vi "ATM_Client.vi"() -> ()   [LabVIEW 2023]
uses:
  Controller/ControllerAccount.ctl
  Controller/ControllerATM.ctl
  Controller/ControllerMenu.ctl
  <vilib>/Utility/error.llb/Trim Whitespace One-Sided.vi
  <vilib>/Utility/file.llb/Read Delimited Spreadsheet (string).vi
  <vilib>/regexp/Match Regular Expression.xnode
panel:
  out "Error reading \nLog.txt":errorcluster
  out "Error reading \nAccounts.txt":errorcluster
  out "Withdrawal Error":errorcluster
  out "Deposit Error":errorcluster
  out "Fast Cash \nWithdrawal Error":errorcluster
  out "Exit Error":errorcluster
  out "Check Balance \nError":errorcluster
  out "Operation \nTimeout Error":errorcluster
  out "Login Timeout Error":errorcluster
  out "Login Error":errorcluster
  in  "Exit Admin Page":bool
  in  "Admin":enum32{"User Details", "Log Acivity"}(tab)
  out "Users":string[][](table)
  out "Log":string[][](table)
  in  "Right Buttons":T1
  out "Right Menu":T2
  out "Left Menu":T3
  in  "Left Buttons":T4
  out "Events":T5
  in  "Account No.":string
  in  "Enter Button":bool
  in  "User Input":string
  in  "Card Simulator":bool
  out "ATM Messages":string
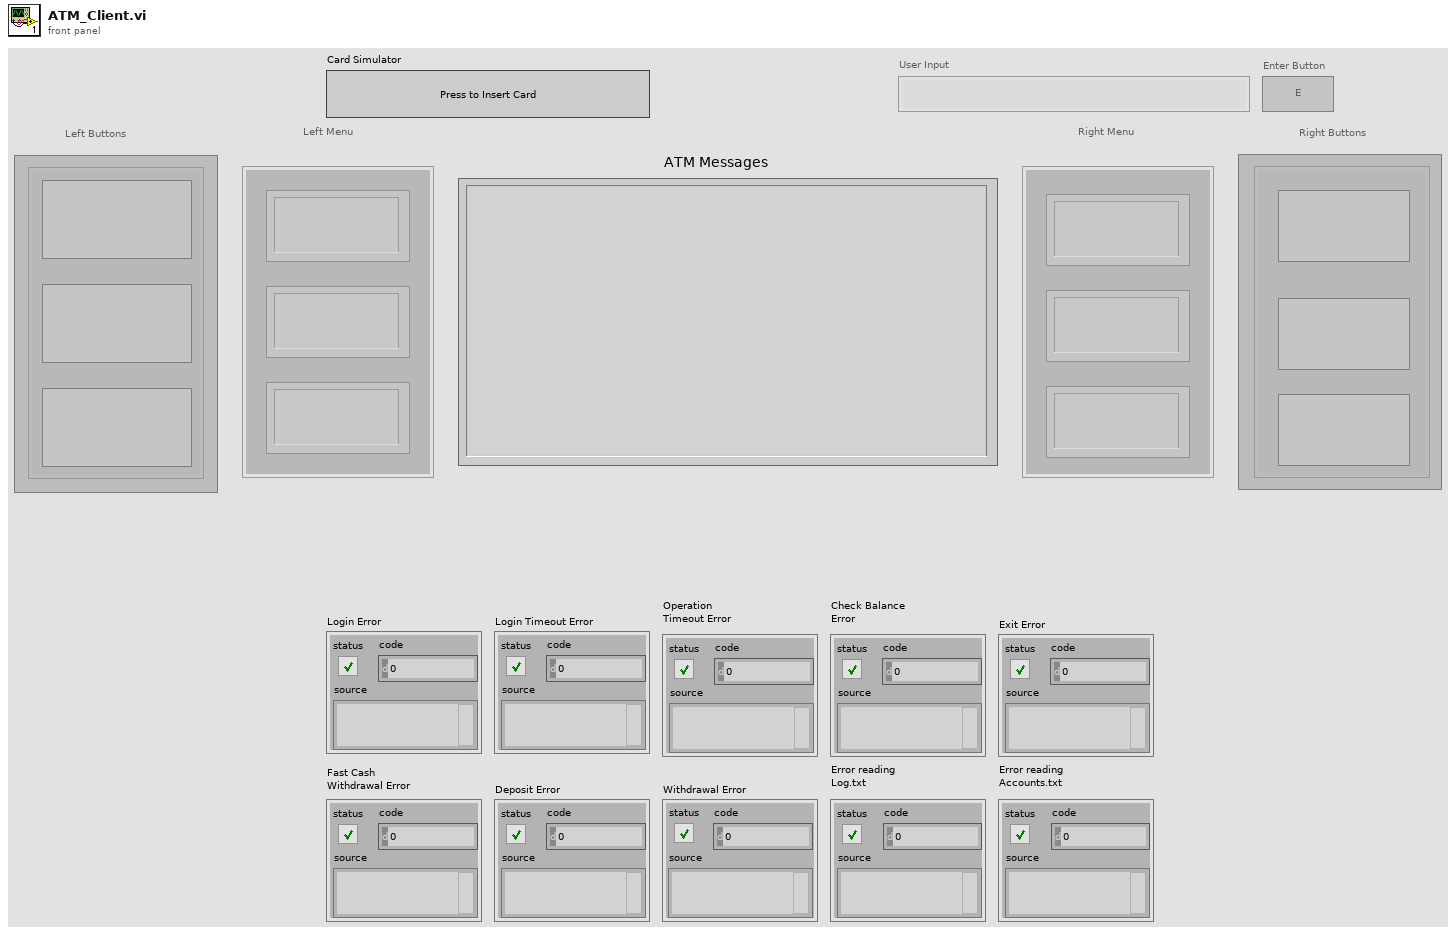
[diagram p1: front panel]
types:
  T1 = cluster{"Right Button 1":bool, "Right Button 2":bool, "Right Button 3":bool}
  T2 = cluster{"Right Menu 1":string, "Right Menu 2":string, "Right Menu 3":string}
  T3 = cluster{"Left Menu 1":string, "Left Menu 2":string, "Left Menu 3":string}
  T4 = cluster{"Left Button 1":bool, "Left Button 2":bool, "Left Button 3":bool}
  T5 = typedef "ControllerAccount.ctl" = enum16{"Deactivate", "Deposit", "Withdraw"}
  T6 = typedef "ControllerATM.ctl" = enum16{"Welcome", "Login", "Main"}
  T7 = enum8{"Enabled", "Disabled", "Disabled and Grayed Out"}
  T8 = typedef "ControllerMenu.ctl" = enum16{"Initialization", "Processes"}
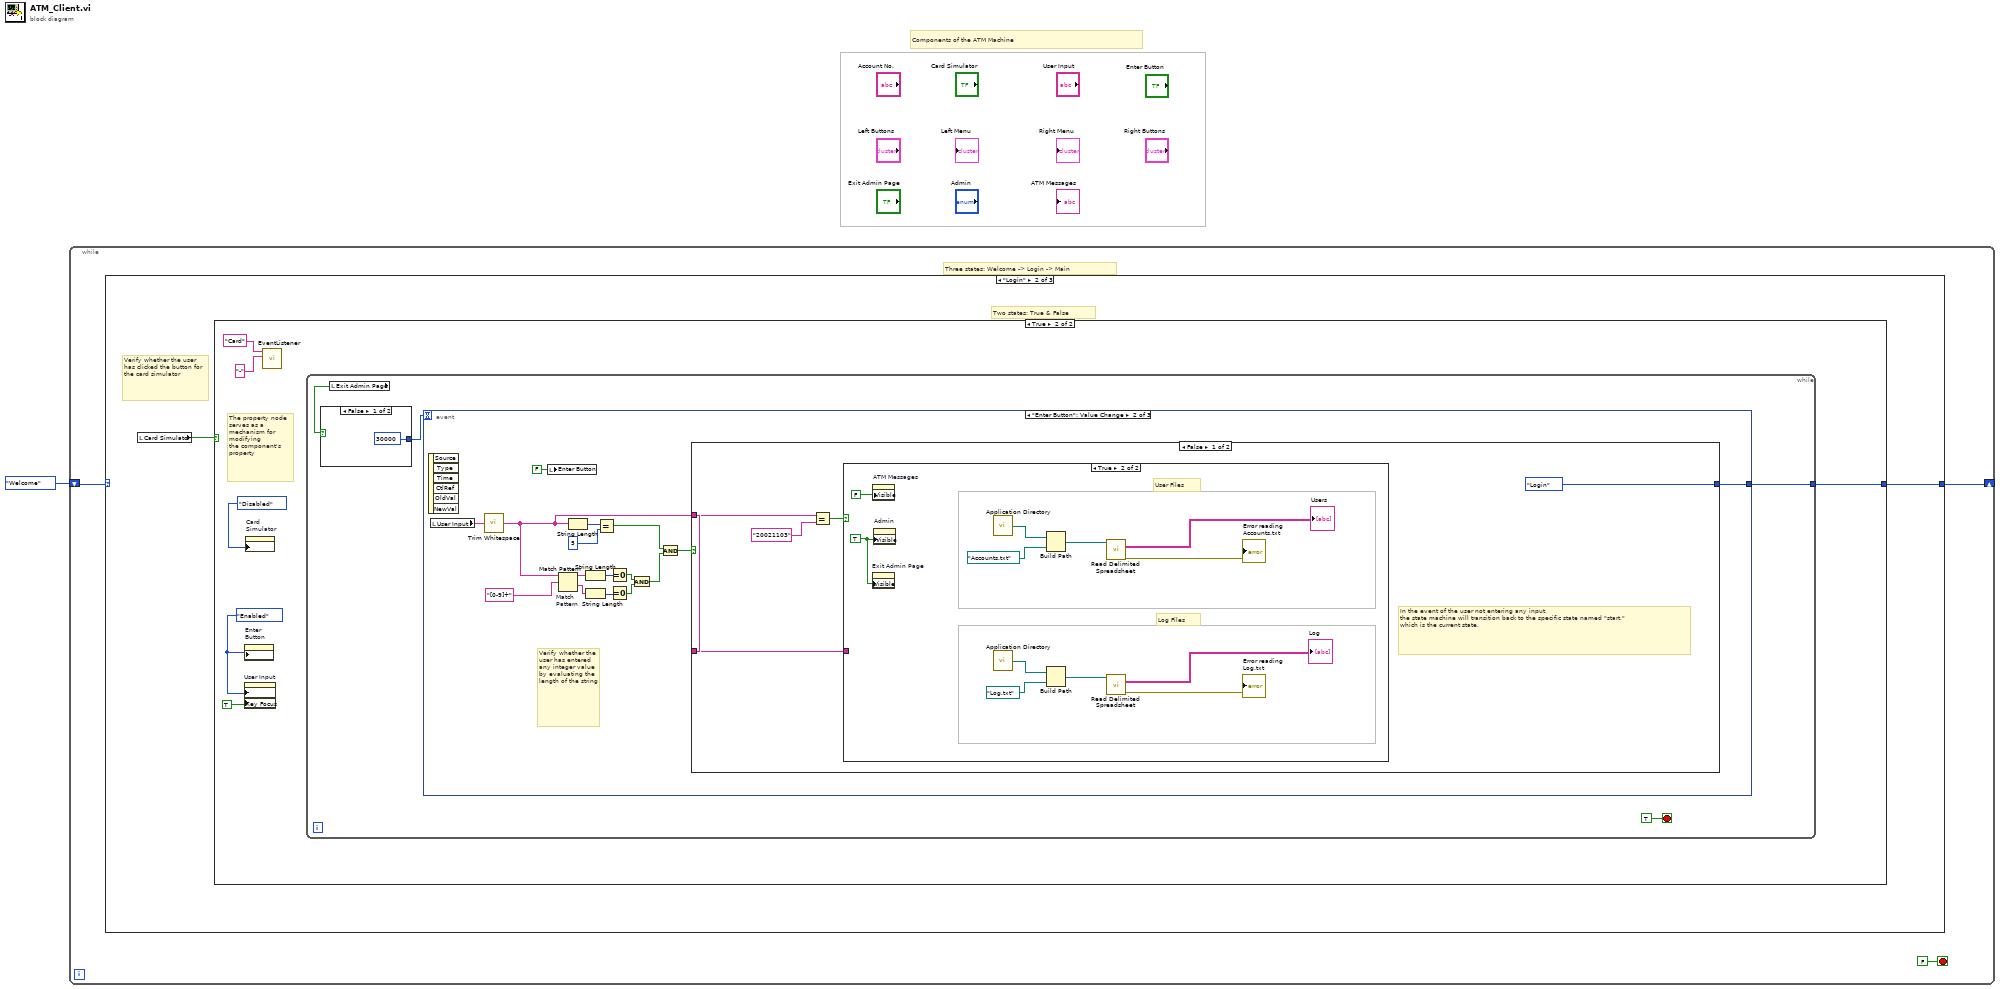
[diagram p0: block diagram]
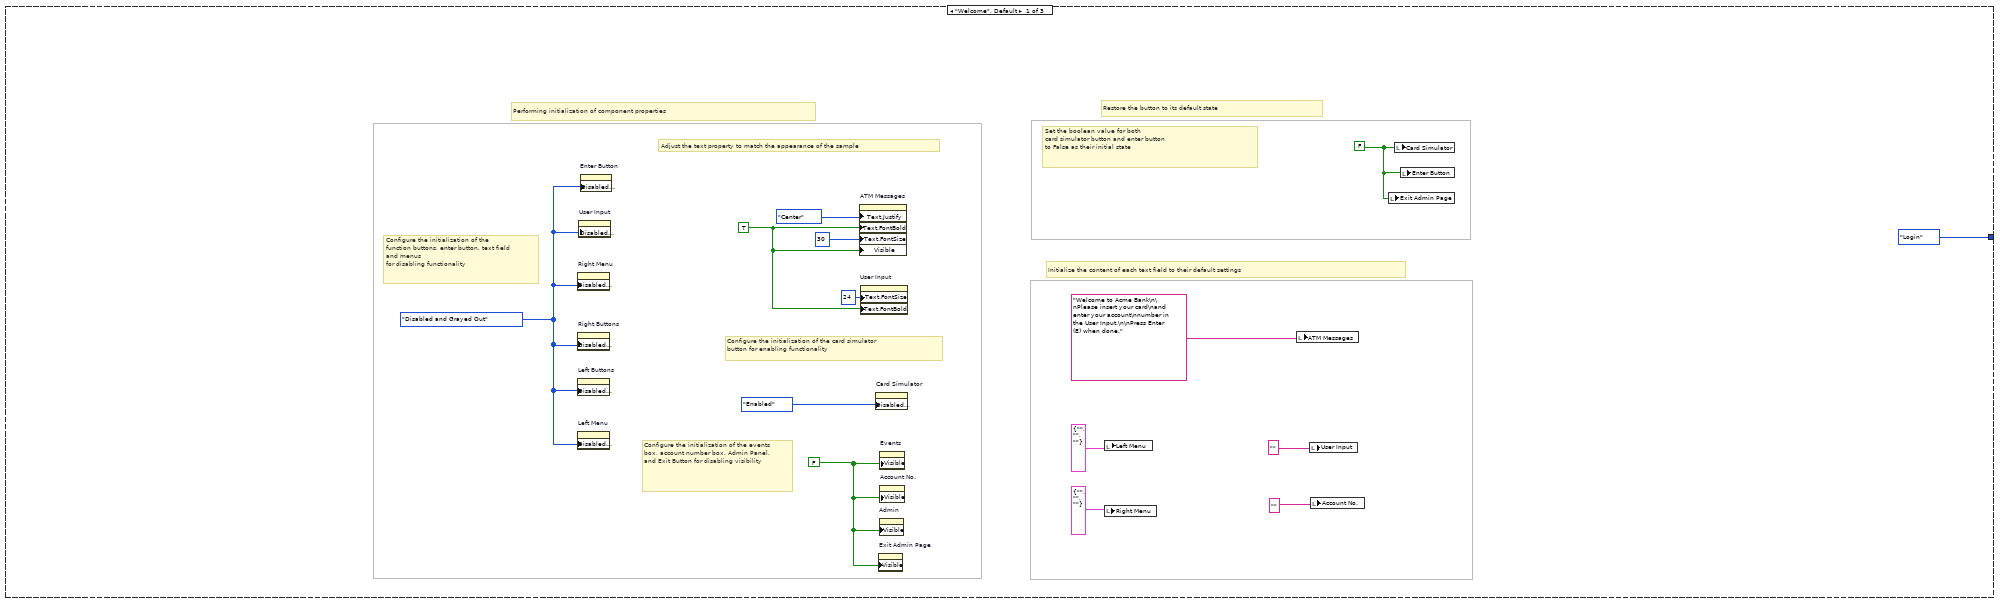
[diagram p2: hidden frame]
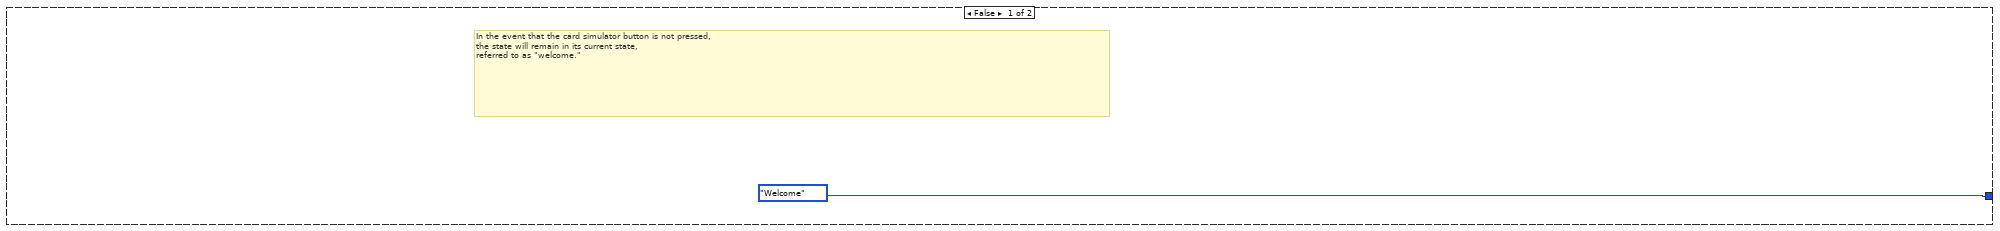
[diagram p3: hidden frame]
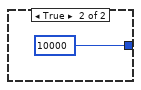
[diagram p4: hidden frame]
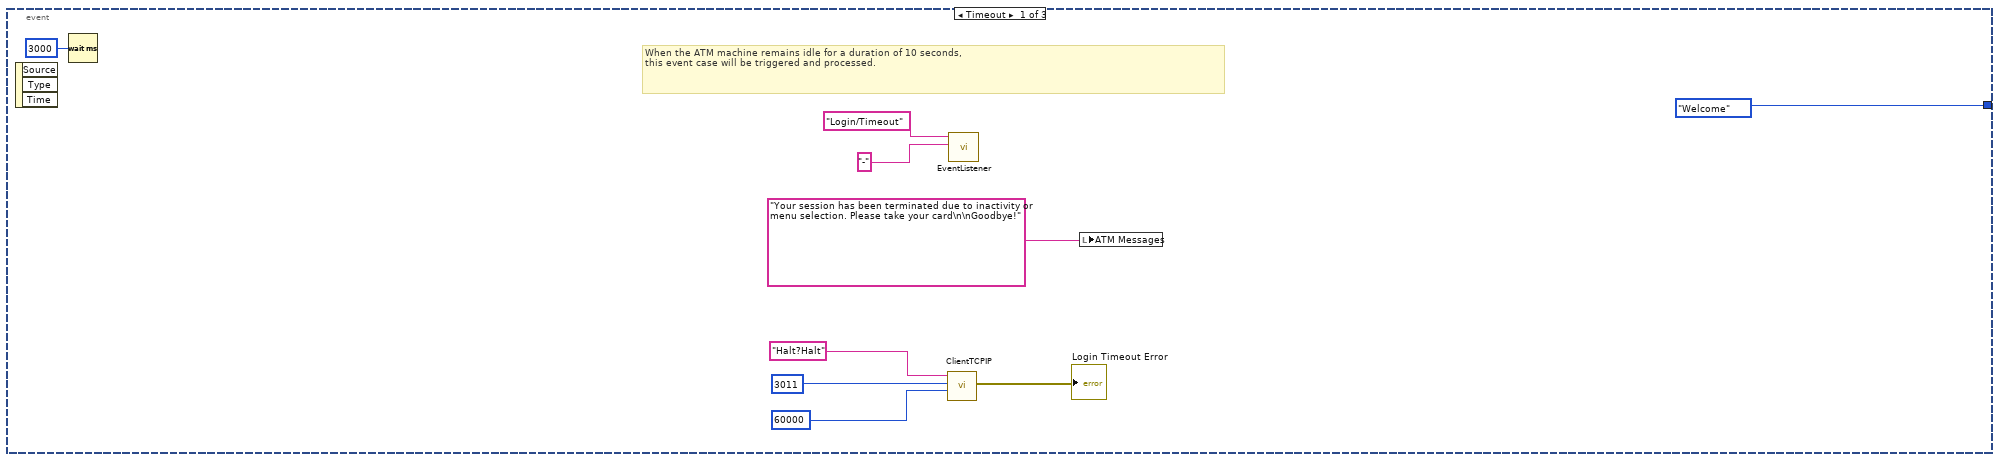
[diagram p5: hidden frame]
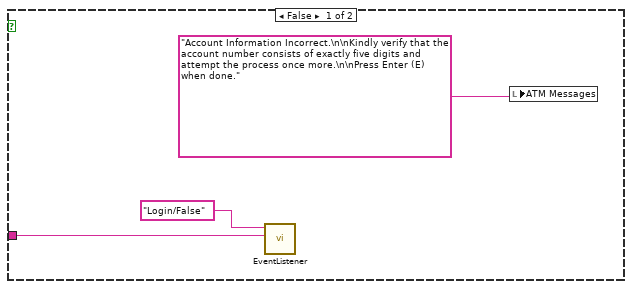
[diagram p6: hidden frame]
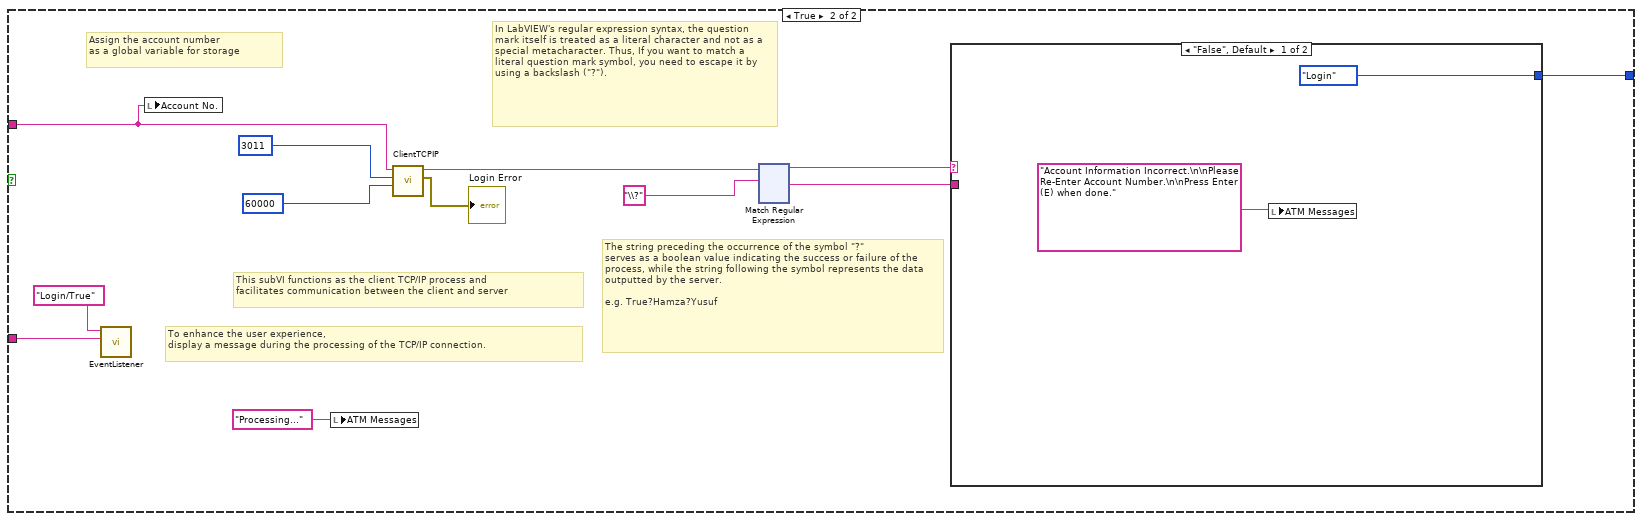
[diagram p7: hidden frame]
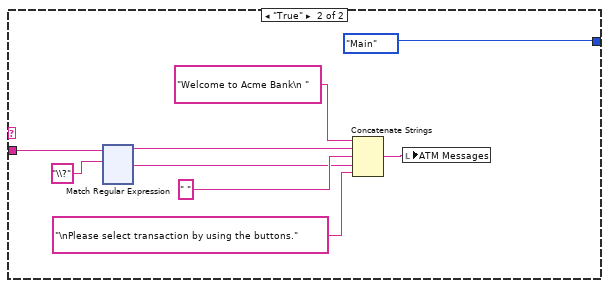
[diagram p8: hidden frame]
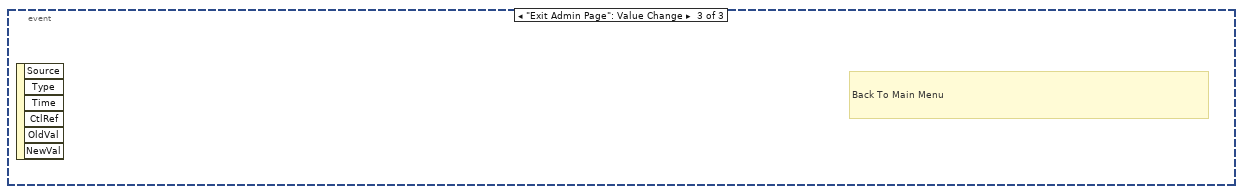
[diagram p9: hidden frame]
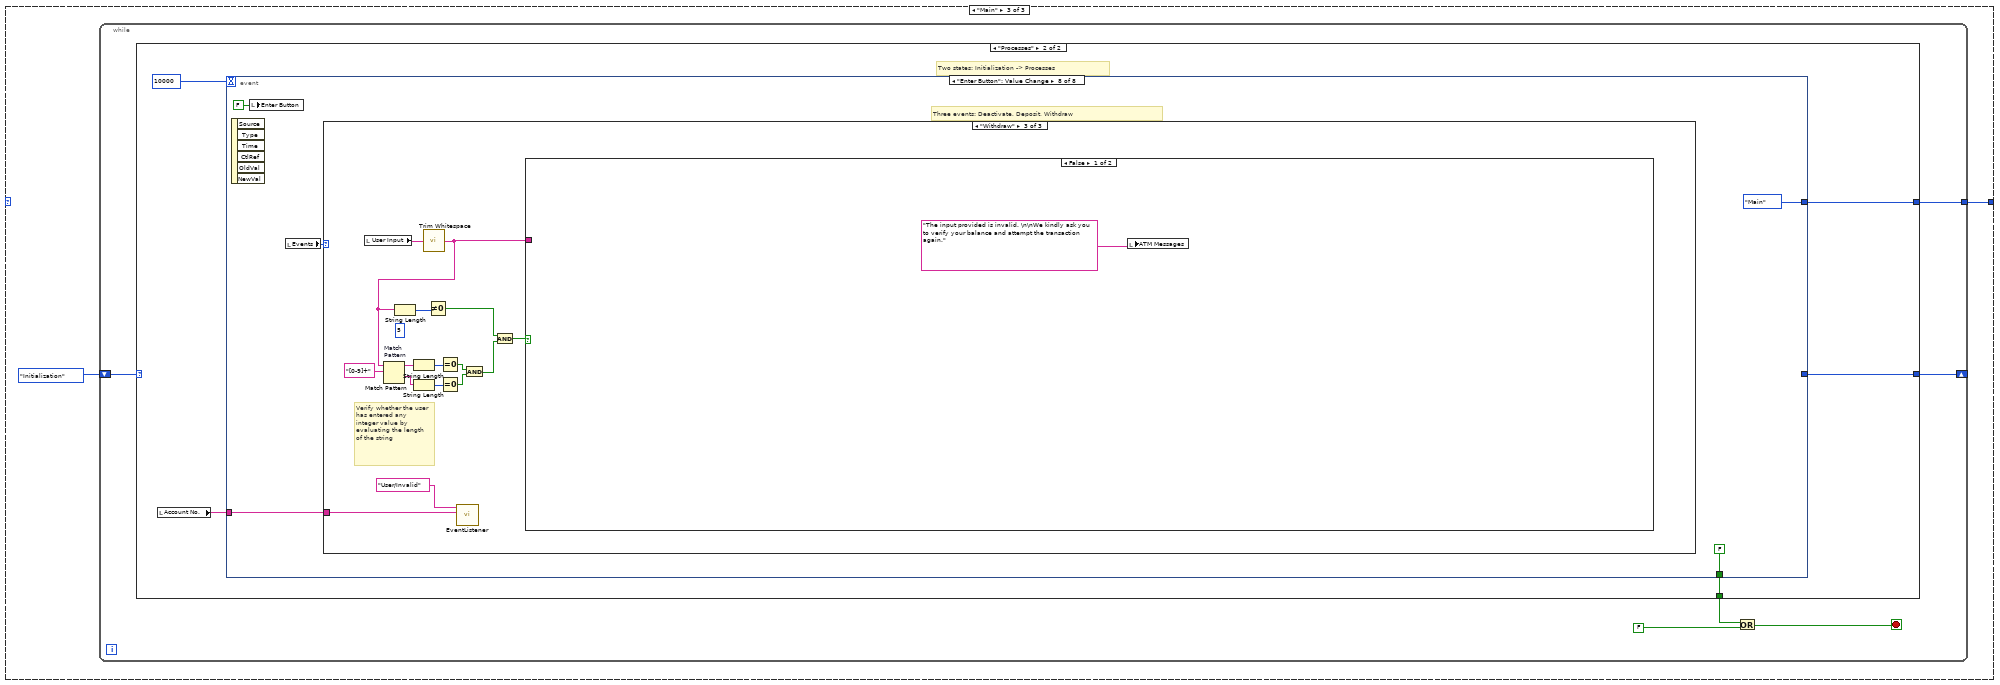
[diagram p10: hidden frame]
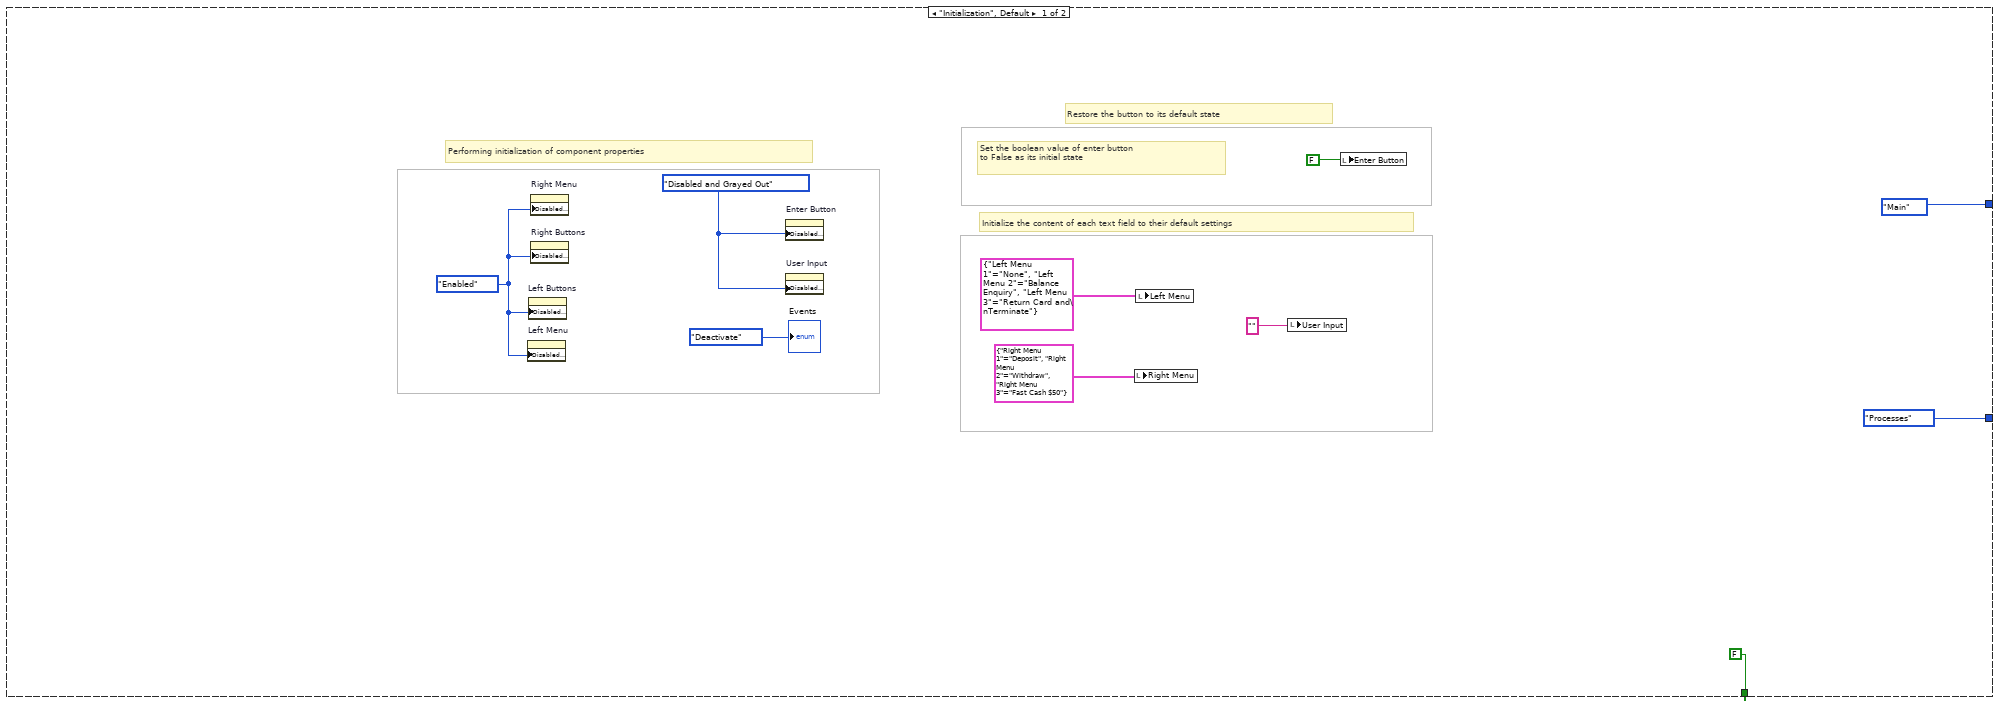
[diagram p11: hidden frame]
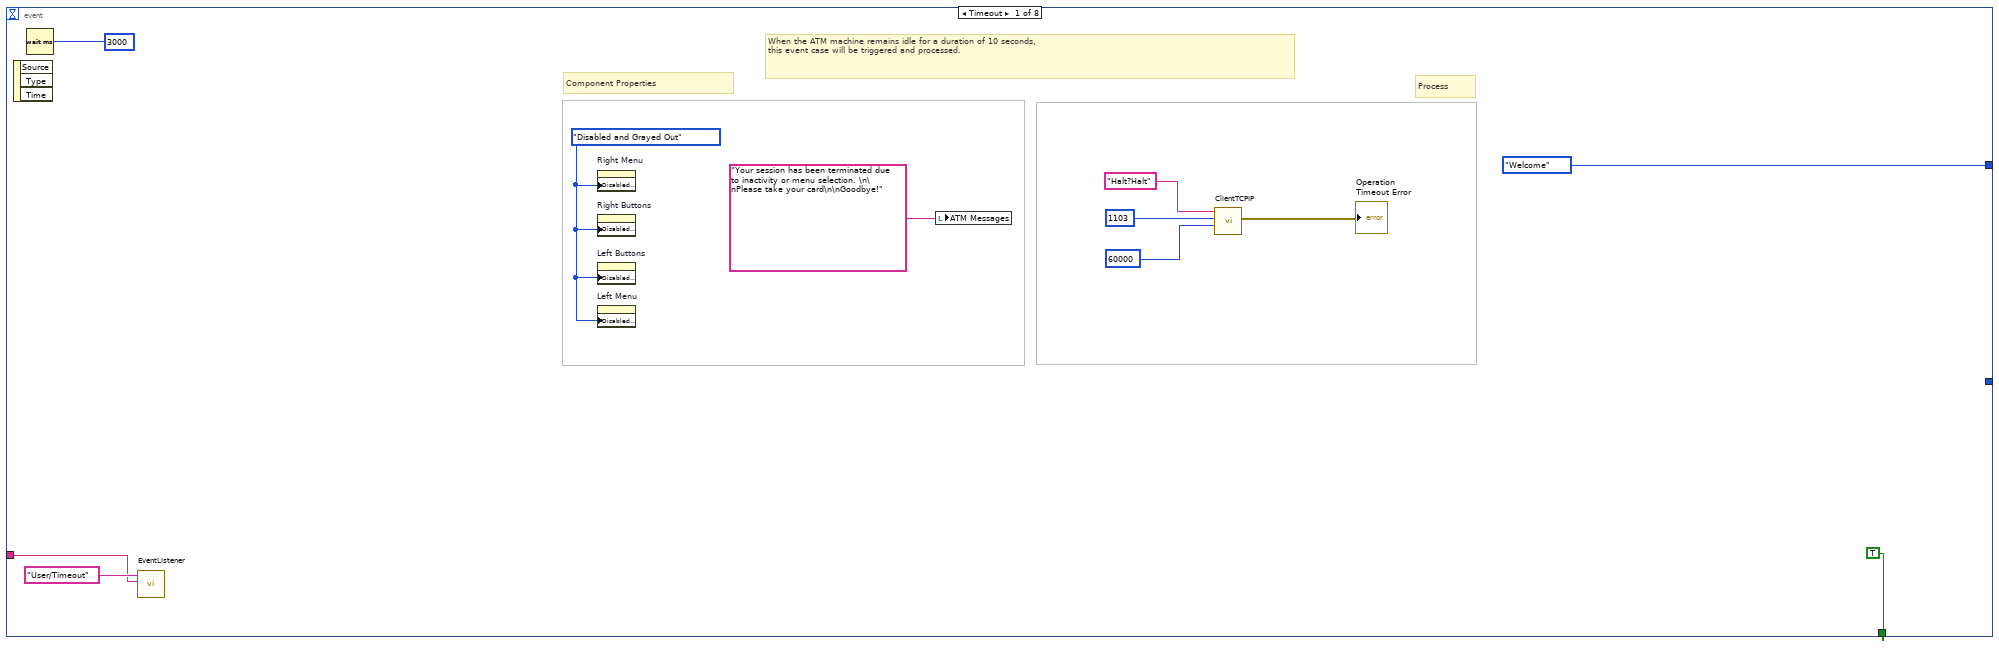
[diagram p12: hidden frame]
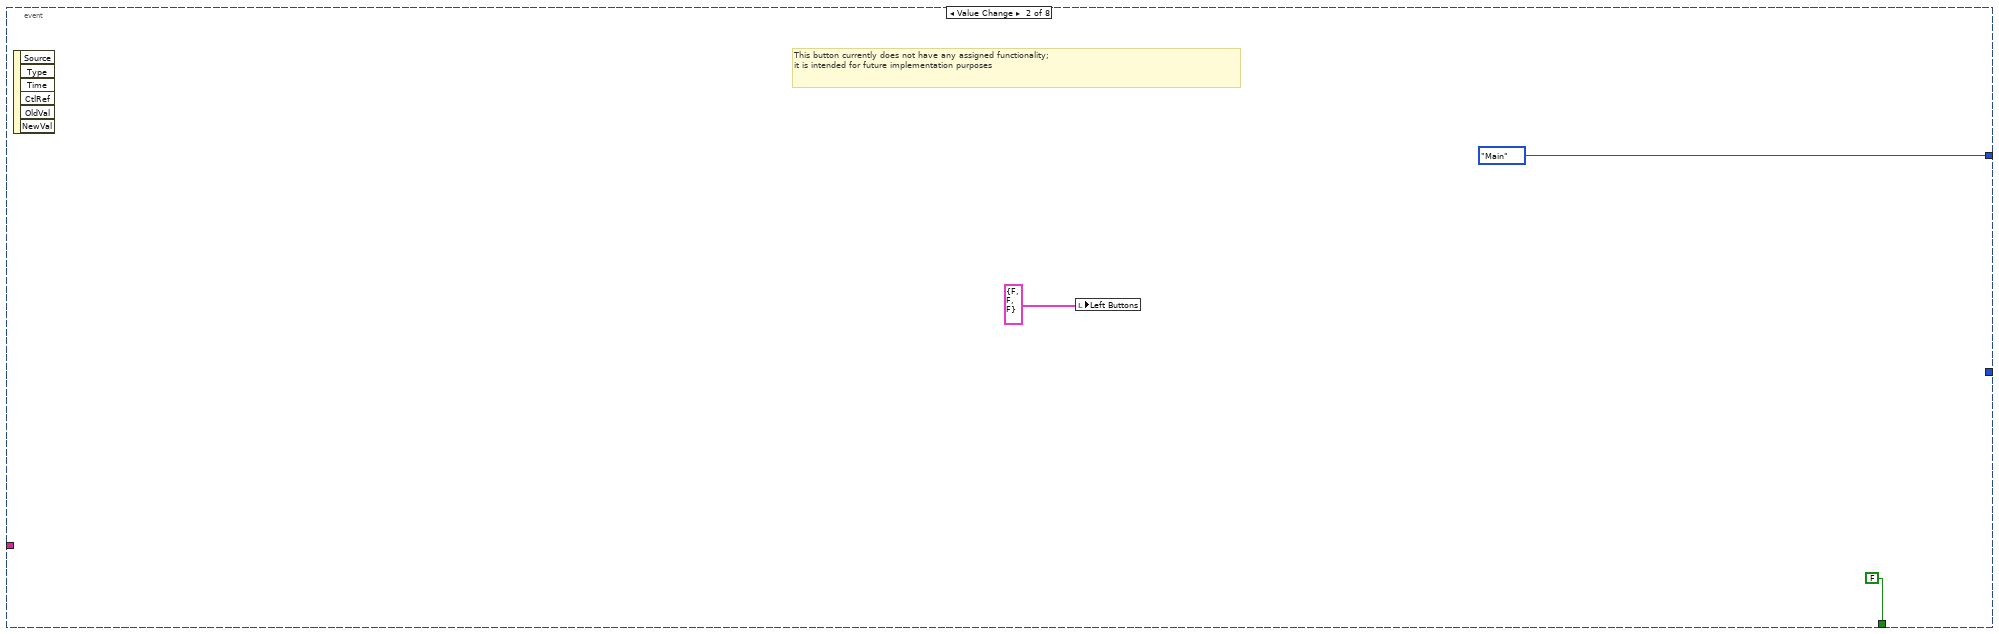
[diagram p13: hidden frame]
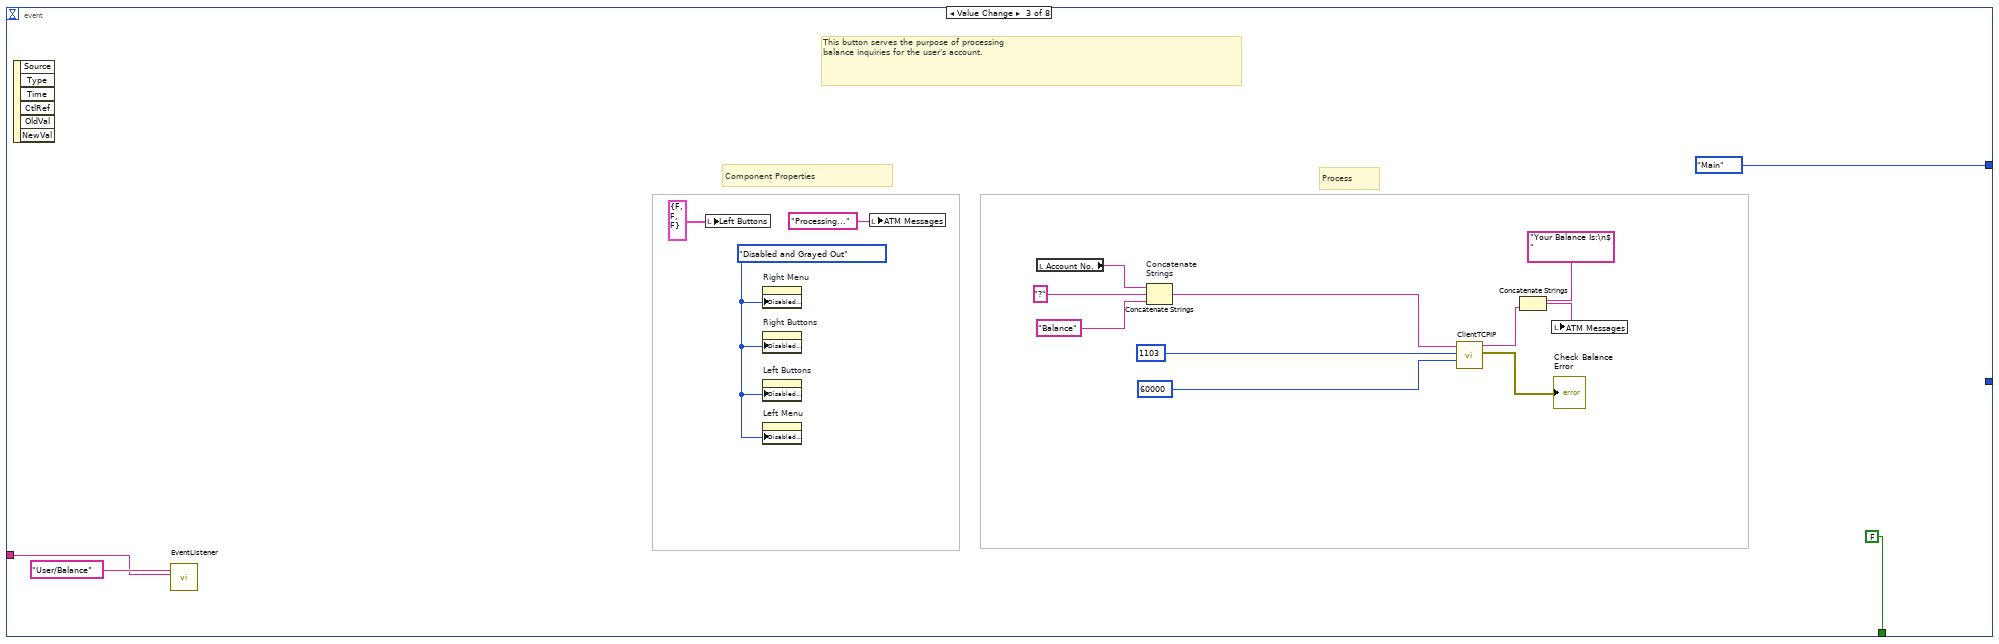
[diagram p14: hidden frame]
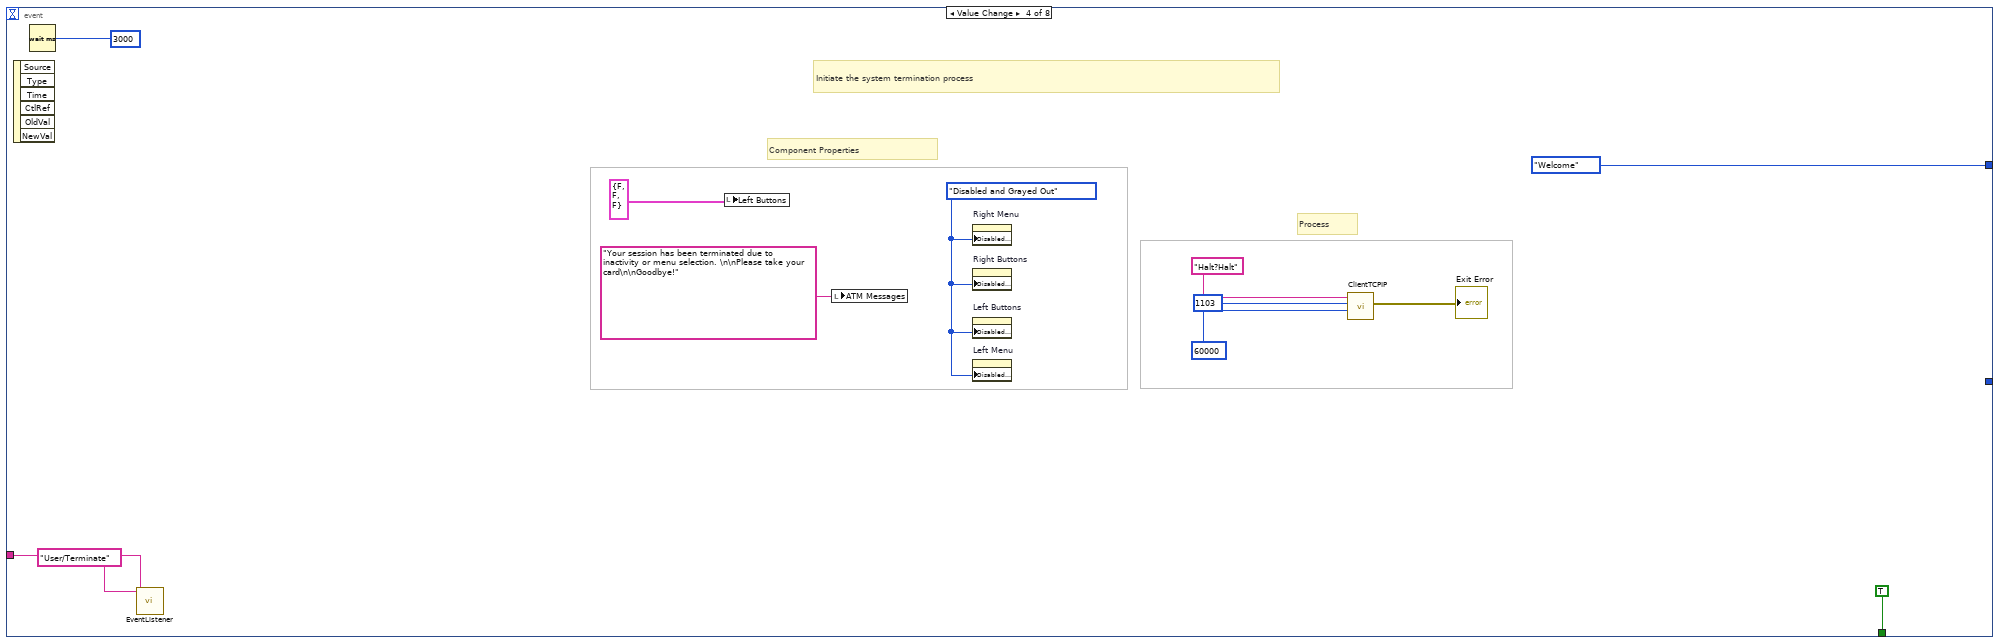
[diagram p15: hidden frame]
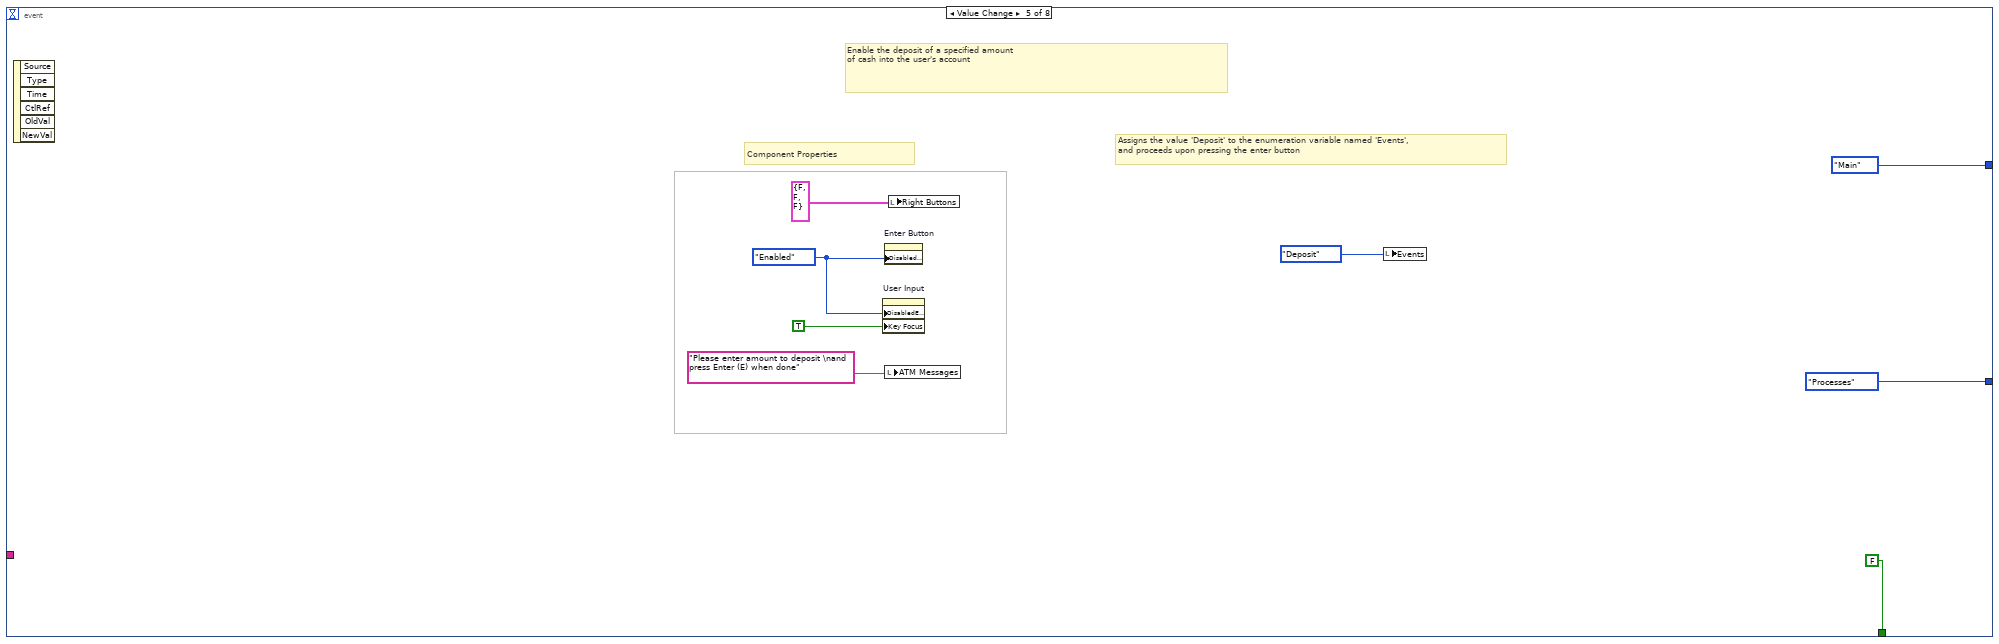
[diagram p16: hidden frame]
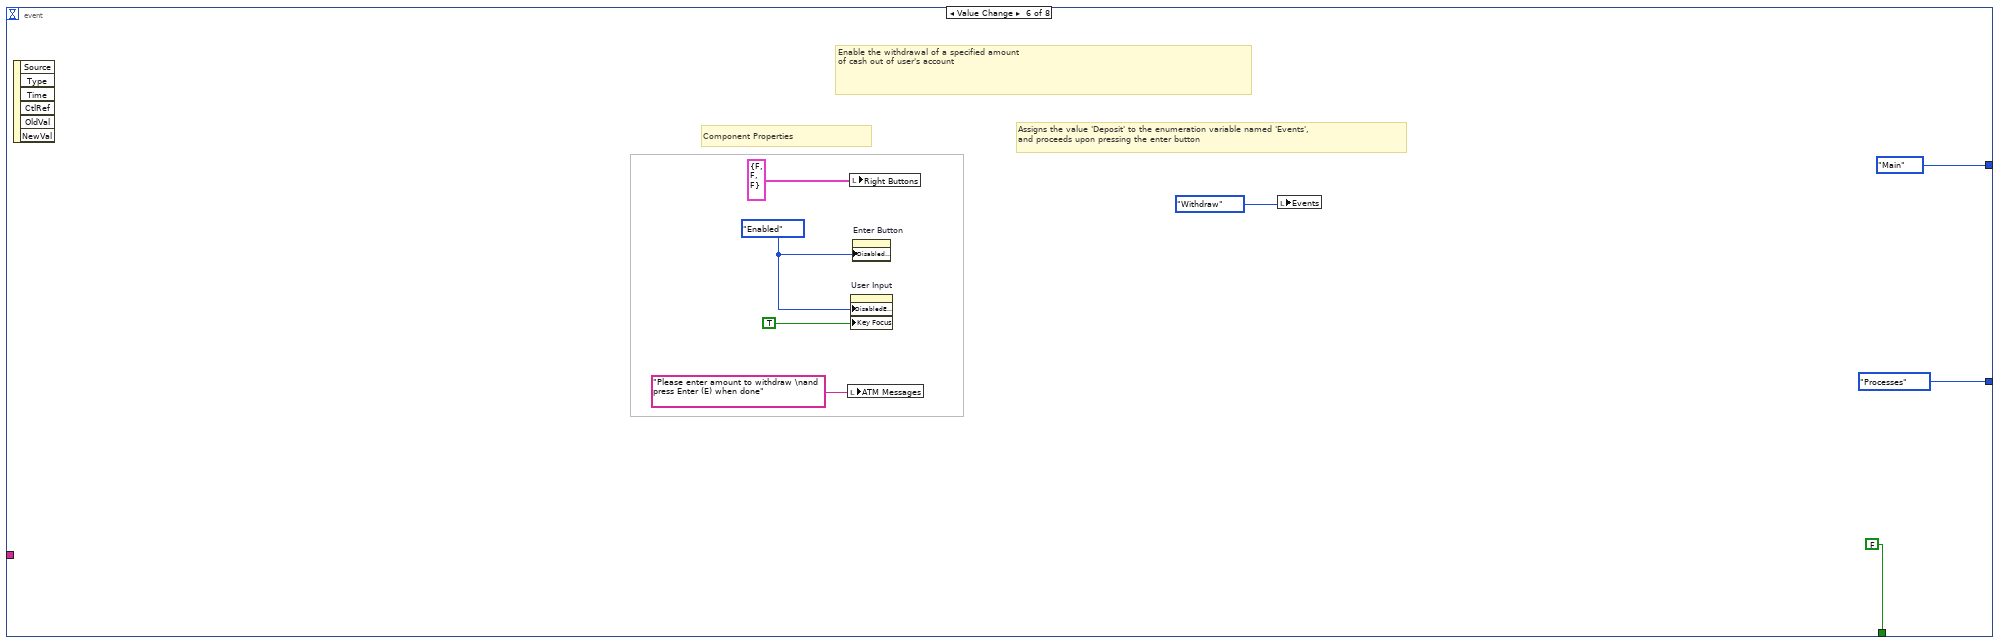
[diagram p17: hidden frame]
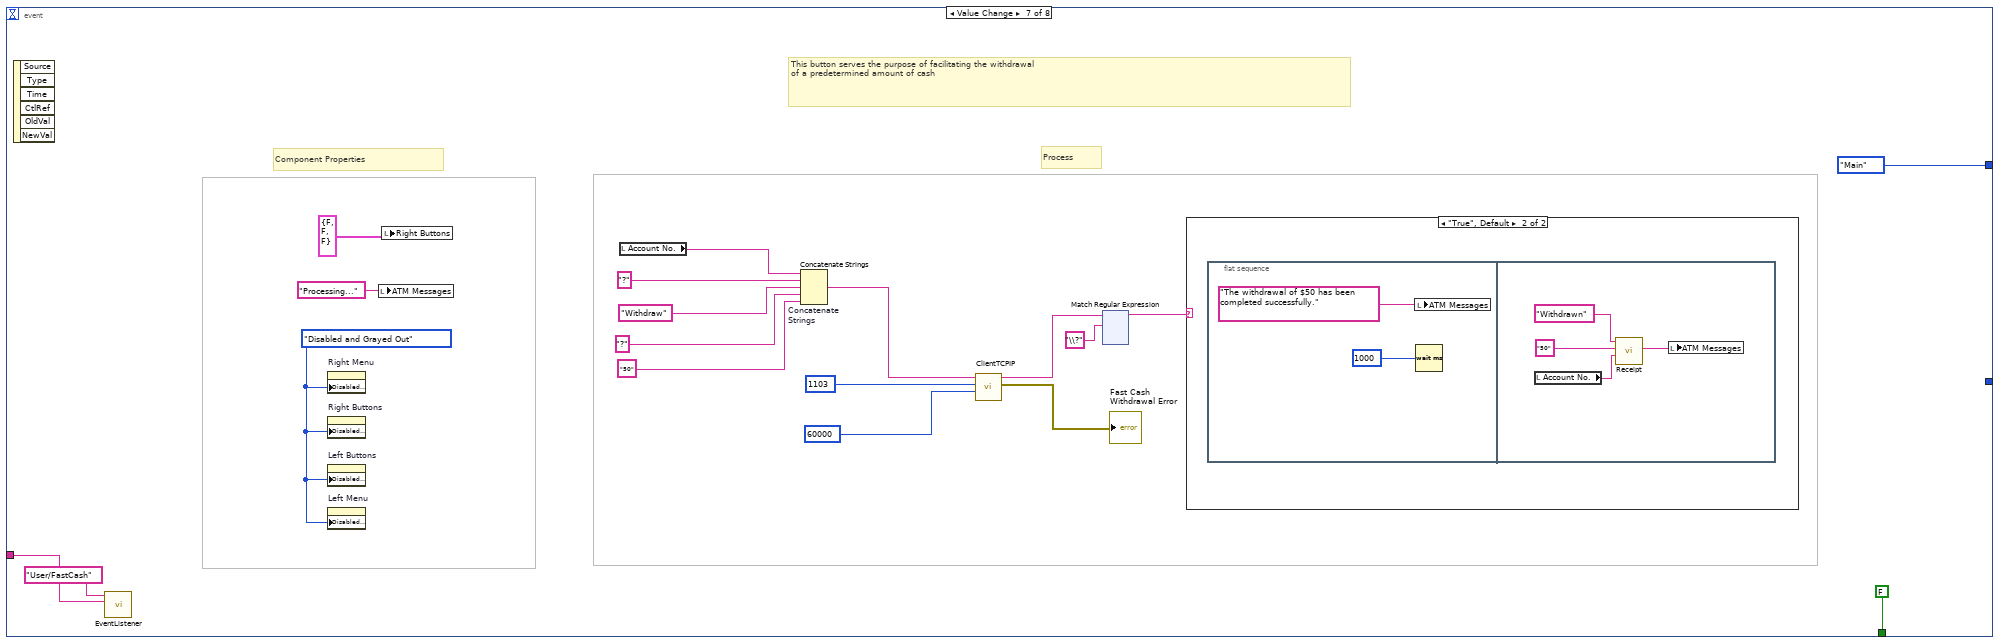
[diagram p18: hidden frame]
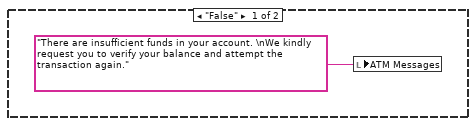
[diagram p19: hidden frame]
diagram:
  # "Components of the ATM Machine"
  n1 = while {
    shift-right: [w3] -> _
    shift-left: ControllerATM."Welcome" ("ATM State") -> [w4]
    stop <- FALSE stop-if-true
    # "Three states: Welcome -> Login -> Main"
    n2 = case shown="\"Login\"" w4 {
      tunnel: [ControllerATM."Login" w19 w336] -> w3
      frame "Welcome", Default {
        w6 = FALSE ("Visible")
        w9 = T7."Disabled and Grayed Out" ("Disabled")
        w7 = TRUE ("Text.Font:Bold")
        w5 = FALSE ("Card Simulator")
        # "Configure the initialization of the events box, account number box, Admin Panel, and Exit Button for disabling visibility"
        # "Initialize the content of each text field to their default settings"
        # "Set the boolean value for both \ncard simulator button and enter button \nto False as their initial state"
        # "Configure the initialization of the \nfunction buttons, enter button, text field and menus \nfor disabling functionality"
        # "Performing initialization of component properties"
        # "Configure the initialization of the card simulator \nbutton for enabling functionality"
        # "Adjust the text property to match the appearance of the sample"
        # "Restore the button to its default state"
        n3 = property on="Right Menu" class="Clust (strict)"("DisabledEnum"=w9) -> ()  [unwired: 2 in, 2 out]
        n4 = property on="Right Buttons" class="Clust (strict)"("DisabledEnum"=w9) -> ()  [unwired: 2 in, 2 out]
        n5 = property on="Left Buttons" class="Clust (strict)"("DisabledEnum"=w9) -> ()  [unwired: 2 in, 2 out]
        n6 = property on="Left Menu" class="Clust (strict)"("DisabledEnum"=w9) -> ()  [unwired: 2 in, 2 out]
        n7 = property on="User Input" class="Str"("DisabledEnum"=w9) -> ()  [unwired: 2 in, 2 out]
        n8 = property on="Enter Button" class="Bool (strict)"("DisabledEnum"=w9) -> ()  [unwired: 2 in, 2 out]
        n9 = property on="ATM Messages" class="Str"("Text.Justify"=enum16{"Left", "Center", "Right"}."Center" ("Text.Justification"), "Text.FontBold"=w7, "Text.FontSize"=u32 30 ("Text.Font:Size"), "Visible"=w7) -> ()  [unwired: 2 in, 2 out]
        n10 = property on="User Input" class="Str"("Text.FontSize"=u32 24 ("Text.Font:Size"), "Text.FontBold"=w7) -> ()  [unwired: 2 in, 2 out]
        n11 = property on="Card Simulator" class="Bool (strict)"("DisabledEnum"=T7."Enabled" ("Disabled")) -> ()  [unwired: 2 in, 2 out]
        n12 = property on="Exit Admin Page" class="Bool (strict)"("Visible"=w6) -> ()  [unwired: 2 in, 2 out]
        n13 = property on="Admin" class="TabCtl (strict)"("Visible"=w6) -> ()  [unwired: 2 in, 2 out]
        n14 = property on="Events" class="Enum (strict)"("Visible"=w6) -> ()  [unwired: 2 in, 2 out]
        n15 = property on="Account No." class="Str"("Visible"=w6) -> ()  [unwired: 2 in, 2 out]
        n16 = local write "Right Menu"(T2 {"Right Menu 1"="", "Right Menu 2"="", "Right Menu 3"=""} ("Right Menu")) -> ()
        n17 = local write "Left Menu"(T3 {"Left Menu 1"="", "Left Menu 2"="", "Left Menu 3"=""} ("Left Menu")) -> ()
        n18 = local write "ATM Messages"("Welcome to Acme Bank\n\nPlease insert your card\nand enter your account\nnumber in the User Input.\n\nPress Enter (E) when done." ("ATM")) -> ()
        n19 = local write "User Input"("" ("User Input")) -> ()
        n20 = local write "Account No."("" ("Account No.")) -> ()
        n21 = local write "Exit Admin Page"(w5) -> ()
        n22 = local write "Card Simulator"(w5) -> ()
        n23 = local write "Enter Button"(w5) -> ()
      }
      frame "Login" {
        # "Two states: True & False"
        # "Verify whether the user has clicked the button for the card simulator"
        n24 = local read "Card Simulator"() -> (w20:bool)
        n25 = case shown="True" w20 {
          tunnel: [ControllerATM."Welcome" w25] -> w19
          frame False {
            # "In the event that the card simulator button is not pressed, \nthe state will remain in its current state, \nreferred to as \"welcome.\""
          }
          frame True {
            w27 = T7."Enabled" ("Disabled")
            # "The property node serves as a mechanism for modifying \nthe component's \nproperty"
            n26 = property on="User Input" class="Str"("DisabledEnum"=w27, "Key Focus"=TRUE) -> ()  [unwired: 2 in, 2 out]
            n27 = property on="Enter \nButton" class="Bool (strict)"("DisabledEnum"=w27) -> ()  [unwired: 2 in, 2 out]
            n28 = property on="Card \nSimulator" class="Bool (strict)"("DisabledEnum"=T7."Disabled" ("Disabled")) -> ()  [unwired: 2 in, 2 out]
            n29 = call "EventListener.vi"("Account No."="-", "Cases"="Card") -> ()  [unwired: 10 in]
            n30 = while {
              tunnel: [w31] -> w25
              stop <- TRUE stop-if-true
              n31 = local read "Exit Admin Page"() -> (w29:bool)
              n32 = case shown="False" w29 {
                tunnel: [30000 10000] -> w28
                frame False {
                }
                frame True {
                }
              }
              n33 = event shown="[1] \"Enter Button\": Value Change" {
                selector: _ -> [_ _ _]
                dyn-events: _ -> [_ _ _]
                timeout: w28 -> [_ _ _]
                tunnel: [ControllerATM."Welcome" w57 _] -> w31
                event Timeout {
                  # "When the ATM machine remains idle for a duration of 10 seconds, \nthis event case will be triggered and processed."
                  n34 = event-data() -> ()  [unwired: 1 in, 3 out]
                  n35 = Wait (ms)(milliseconds to wait=u32 3000) -> ()  [unwired: 1 out]
                  n36 = call "ClientTCPIP.vi"("timeout \nms (60000)"=60000 ("timeout ms (60000)"), "port"=u16 3011 ("remote port or service name"), "Input String"="Halt?Halt" ("data in")) -> ("error out"=→"Login Timeout Error":errorcluster)  [unwired: 7 in, 1 out]
                  n37 = call "EventListener.vi"("Account No."="-", "Cases"="Login/Timeout") -> ()  [unwired: 10 in]
                  n38 = local write "ATM Messages"("Your session has been terminated due to inactivity or menu selection. Please take your card\n\nGoodbye!" ("ATM")) -> ()
                }
                event "Enter Button": Value Change {
                  # "Verify whether the user has entered any integer value by evaluating the length of the string"
                  n39 = event-data() -> ()  [unwired: 1 in, 6 out]
                  n40 = local read "User Input"() -> (w45:string)
                  n41 = call <vilib>:"Trim Whitespace.vi"("string"=w45) -> ("trimmed string"=w43:string)  [unwired: 1 in]
                  n42 = local write "Enter Button"(FALSE ("Enter Button")) -> ()
                  n43 = Match Pattern "Match \nPattern"(string=w43, regular expression="[0-9]+") -> (before substring=w51:string, after substring=w52:string)  [unwired: 1 in, 2 out]
                  n44 = String Length(string=w43) -> (length=w48:i32)
                  n45 = String Length(string=w51) -> (length=w49:i32)
                  n46 = String Length(string=w52) -> (length=w50:i32)
                  n47 = Equal?(x=w48, y=5) -> (x = y?=w56:bool)
                  n48 = Equal To 0?(x=w49) -> (x = 0?=w53:bool)
                  n49 = Equal To 0?(x=w50) -> (x = 0?=w54:bool)
                  n50 = And(x=w53, y=w54) -> (x .and. y?=w55:bool)
                  n51 = And(x=w56, y=w55) -> (x .and. y?=w44:bool)
                  n52 = case shown="False" w44 {
                    tunnel: [ControllerATM."Login" w87] -> w57
                    tunnel: w43 -> [w60 w81]
                    tunnel: w43 -> [w59 w80]
                    frame False {
                      # "In the event of the user not entering any input, \nthe state machine will transition back to the specific state named \"start,\" \nwhich is the current state."
                      n53 = Equal?(x=w60, y="20021103") -> (x = y?=w61:bool)
                      n54 = case shown="True" w61 {
                        tunnel: w59 -> [w64 _]
                        frame False {
                          n55 = call "EventListener.vi"("Account No."=w64, "Cases"="Login/False") -> ()  [unwired: 10 in]
                          n56 = local write "ATM Messages"("Account Information Incorrect.\n\nKindly verify that the account number consists of exactly five digits and attempt the process once more.\n\nPress Enter (E) when done." ("ATM")) -> ()
                        }
                        frame True {
                          w78 = TRUE ("Visible")
                          # "Log Files"
                          # "User Files"
                          n57 = property on="Exit Admin Page" class="Bool (strict)"("Visible"=w78) -> ()  [unwired: 2 in, 2 out]
                          n58 = property on="ATM Messages" class="Str"("Visible"=FALSE) -> ()  [unwired: 2 in, 2 out]
                          n59 = property on="Admin" class="TabCtl (strict)"("Visible"=w78) -> ()  [unwired: 2 in, 2 out]
                          n60 = call <vilib>:"Application Directory.vi"() -> ("Application Directory"=w74:path)
                          n61 = call <vilib>:"Application Directory.vi"() -> ("Application Directory"=w71:path)
                          n62 = Build Path(base path=w74, name or relative path=path "Accounts.txt") -> (appended path=w75:path)
                          n63 = Build Path(base path=w71, name or relative path=path "Log.txt") -> (appended path=w70:path)
                          n64 = call-poly <vilib>:"Read Delimited Spreadsheet.vi"("file path (dialog if empty)"=w75) -> ("all rows"=→"Users":string[][], "error out"=→"Error reading \nAccounts.txt":errorcluster)  [unwired: 9 in, 4 out]
                          n65 = call-poly <vilib>:"Read Delimited Spreadsheet.vi"("file path (dialog if empty)"=w70) -> ("all rows"=→"Log":string[][], "error out"=→"Error reading \nLog.txt":errorcluster)  [unwired: 9 in, 4 out]
                        }
                      }
                    }
                    frame True {
                      # "In LabVIEW's regular expression syntax, the question mark itself is treated as a literal character and not as a special metacharacter. Thus, If you want to match a literal question mark symbol, you need to escape it by using a backslash (\"?\")."
                      # "The string preceding the occurrence of the symbol \"?\" \nserves as a boolean value indicating the success or failure of the process, while the string following the symbol represents the data outputted by the server.\n\ne.g. True?Hamza?Yusuf"
                      # "This subVI functions as the client TCP/IP process and \nfacilitates communication between the client and server"
                      # "To enhance the user experience, \ndisplay a message during the processing of the TCP/IP connection."
                      # "Assign the account number \nas a global variable for storage"
                      n66 = call "EventListener.vi"("Account No."=w80, "Cases"="Login/True") -> ()  [unwired: 10 in]
                      n67 = local write "Account No."(w81) -> ()
                      n68 = local write "ATM Messages"("Processing..." ("ATM Messages")) -> ()
                      n69 = call "ClientTCPIP.vi"("timeout \nms (60000)"=60000 ("timeout ms (60000)"), "port"=u16 3011 ("remote port or service name"), "Input String"=w81) -> ("error out"=→"Login Error":errorcluster, "Output Data"=w82:string)  [unwired: 7 in]
                      n70 = xnode "Match Regular \nExpression"("input string"=w82, "regular expression"="\\?") -> ("before match"=w88:string, "after match"=w89:string)  [unwired: 4 in, 3 out]
                      n71 = case shown="\"False\", Default" w88 {
                        tunnel: w89 -> [_ w218]
                        tunnel: [ControllerATM."Login" ControllerATM."Main"] -> w87
                        frame "False", Default {
                          n72 = local write "ATM Messages"("Account Information Incorrect.\n\nPlease Re-Enter Account Number.\n\nPress Enter (E) when done." ("ATM")) -> ()
                        }
                        frame "True" {
                          n73 = xnode "Match Regular Expression"("input string"=w218, "regular expression"="\\?") -> ("before match"=w216:string, "after match"=w213:string)  [unwired: 4 in, 3 out]
                          n74 = Concatenate Strings("Welcome to Acme Bank\n " ("string"), w216, " " ("string"), w213, "\nPlease select transaction by using the buttons." ("string")) -> (w211:string)
                          n75 = local write "ATM Messages"(w211) -> ()
                        }
                      }
                    }
                  }
                }
                event "Exit Admin Page": Value Change {
                  # "Back To Main Menu"
                  n76 = event-data() -> ()  [unwired: 1 in, 6 out]
                }
              }
            }
          }
        }
      }
      frame "Main" {
        n77 = while {
          tunnel: [w339] -> w336
          shift-right: [w338] -> _
          shift-left: ControllerMenu."Initialization" -> [w343]
          stop <- w340 stop-if-true
          n78 = case shown="\"Processes\"" w343 {
            tunnel: [FALSE w356] -> w342
            tunnel: [ControllerATM."Main" w357] -> w339
            tunnel: [ControllerMenu."Processes" w355] -> w338
            frame "Initialization", Default {
              w344 = T7."Enabled" ("Disabled")
              w353 = T7."Disabled and Grayed Out" ("Disabled")
              # "Initialize the content of each text field to their default settings"
              # "Set the boolean value of enter button \nto False as its initial state"
              # "Restore the button to its default state"
              # "Performing initialization of component properties"
              n79 = property on="Left Menu" class="Clust (strict)"("DisabledEnum"=w344) -> ()  [unwired: 2 in, 2 out]
              n80 = property on="Left Buttons" class="Clust (strict)"("DisabledEnum"=w344) -> ()  [unwired: 2 in, 2 out]
              n81 = property on="Right Menu" class="Clust (strict)"("DisabledEnum"=w344) -> ()  [unwired: 2 in, 2 out]
              n82 = property on="Right Buttons" class="Clust (strict)"("DisabledEnum"=w344) -> ()  [unwired: 2 in, 2 out]
              n83 = property on="Enter Button" class="Bool (strict)"("DisabledEnum"=w353) -> ()  [unwired: 2 in, 2 out]
              n84 = property on="User Input" class="Str"("DisabledEnum"=w353) -> ()  [unwired: 2 in, 2 out]
              n85 = local write "Right Menu"(T2 {"Right Menu 1"="Deposit", "Right Menu 2"="Withdraw", "Right Menu 3"="Fast Cash $50"} ("Right Menu")) -> ()
              n86 = local write "Left Menu"(T3 {"Left Menu 1"="None", "Left Menu 2"="Balance Enquiry", "Left Menu 3"="Return Card and\nTerminate"} ("Left Menu")) -> ()
              n87 = local write "User Input"("" ("User Input")) -> ()
              n88 = local write "Enter Button"(FALSE ("Enter Button")) -> ()
              "Events" <- ControllerAccount."Deactivate" ("Enter")
            }
            frame "Processes" {
              # "Two states: Initialization -> Processes"
              n89 = local read "Account No."() -> (w354:string)
              n90 = event shown="[7] \"Enter Button\": Value Change" {
                selector: _ -> [_ _ _ _ _ _ _ _]
                dyn-events: _ -> [_ _ _ _ _ _ _ _]
                timeout: 10000 -> [_ _ _ _ _ _ _ _]
                tunnel: [ControllerATM."Welcome" ControllerATM."Main" ControllerATM."Main" ControllerATM."Welcome" ControllerATM."Main" ControllerATM."Main" ControllerATM."Main" ControllerATM."Main"] -> w357
                tunnel: [TRUE FALSE FALSE TRUE FALSE FALSE FALSE FALSE] -> w356
                tunnel: [_ _ _ _ ControllerMenu."Processes" ControllerMenu."Processes" _ _] -> w355
                tunnel: w354 -> [w359 _ w373 w391 _ _ w419 w561]
                event Timeout {
                  w361 = T7."Disabled and Grayed Out" ("Disabled")
                  # "Process"
                  # "Component Properties"
                  # "When the ATM machine remains idle for a duration of 10 seconds, \nthis event case will be triggered and processed."
                  n91 = event-data() -> ()  [unwired: 1 in, 3 out]
                  n92 = Wait (ms)(milliseconds to wait=u32 3000 ("millisecond timer value")) -> ()  [unwired: 1 out]
                  n93 = call "EventListener.vi"("Account No."=w359, "Cases"="User/Timeout") -> ()  [unwired: 10 in]
                  n94 = property on="Right Menu" class="Clust (strict)"("DisabledEnum"=w361) -> ()  [unwired: 2 in, 2 out]
                  n95 = property on="Right Buttons" class="Clust (strict)"("DisabledEnum"=w361) -> ()  [unwired: 2 in, 2 out]
                  n96 = property on="Left Buttons" class="Clust (strict)"("DisabledEnum"=w361) -> ()  [unwired: 2 in, 2 out]
                  n97 = property on="Left Menu" class="Clust (strict)"("DisabledEnum"=w361) -> ()  [unwired: 2 in, 2 out]
                  n98 = local write "ATM Messages"("Your session has been terminated due to inactivity or menu selection. \n\nPlease take your card\n\nGoodbye!" ("ATM")) -> ()
                  n99 = call "ClientTCPIP.vi"("timeout \nms (60000)"=60000 ("timeout ms (60000)"), "port"=u16 1103 ("remote port or service name"), "Input String"="Halt?Halt" ("data in")) -> ("error out"=→"Operation \nTimeout Error":errorcluster)  [unwired: 7 in, 1 out]
                }
                event "Left Buttons.Left Button 1": Value Change {
                  # "This button currently does not have any assigned functionality; \nit is intended for future implementation purposes"
                  n100 = event-data() -> ()  [unwired: 1 in, 6 out]
                  n101 = local write "Left Buttons"(T4 {"Left Button 1"=FALSE, "Left Button 2"=FALSE, "Left Button 3"=FALSE} ("Left Buttons")) -> ()
                }
                event "Left Buttons.Left Button 2": Value Change {
                  w375 = T7."Disabled and Grayed Out" ("Disabled")
                  # "This button serves the purpose of processing \nbalance inquiries for the user's account."
                  # "Process"
                  # "Component Properties"
                  n102 = event-data() -> ()  [unwired: 1 in, 6 out]
                  n103 = call "EventListener.vi"("Account No."=w373, "Cases"="User/Balance") -> ()  [unwired: 10 in]
                  n104 = local write "Left Buttons"(T4 {"Left Button 1"=FALSE, "Left Button 2"=FALSE, "Left Button 3"=FALSE} ("Left Buttons")) -> ()
                  n105 = property on="Right Menu" class="Clust (strict)"("DisabledEnum"=w375) -> ()  [unwired: 2 in, 2 out]
                  n106 = property on="Right Buttons" class="Clust (strict)"("DisabledEnum"=w375) -> ()  [unwired: 2 in, 2 out]
                  n107 = property on="Left Buttons" class="Clust (strict)"("DisabledEnum"=w375) -> ()  [unwired: 2 in, 2 out]
                  n108 = property on="Left Menu" class="Clust (strict)"("DisabledEnum"=w375) -> ()  [unwired: 2 in, 2 out]
                  n109 = local write "ATM Messages"("Processing..." ("ATM Messages")) -> ()
                  n110 = local read "Account No."() -> (w389:string)
                  n111 = Concatenate Strings "Concatenate \nStrings"(w389, "?" ("string"), "Balance" ("string")) -> (w381:string)
                  n112 = call "ClientTCPIP.vi"("timeout \nms (60000)"=60000 ("timeout ms (60000)"), "port"=u16 1103 ("remote port or service name"), "Input String"=w381) -> ("error out"=→"Check Balance \nError":errorcluster, "Output Data"=w378:string)  [unwired: 7 in]
                  n113 = Concatenate Strings("Your Balance Is:\n$ " ("string"), w378) -> (w386:string)
                  n114 = local write "ATM Messages"(w386) -> ()
                }
                event "Left Buttons.Left Button 3": Value Change {
                  w392 = T7."Disabled and Grayed Out" ("Disabled")
                  # "Initiate the system termination process"
                  # "Process"
                  # "Component Properties"
                  n115 = event-data() -> ()  [unwired: 1 in, 6 out]
                  n116 = Wait (ms)(milliseconds to wait=u32 3000 ("millisecond timer value")) -> ()  [unwired: 1 out]
                  n117 = call "EventListener.vi"("Account No."=w391, "Cases"="User/Terminate") -> ()  [unwired: 10 in]
                  n118 = local write "Left Buttons"(T4 {"Left Button 1"=FALSE, "Left Button 2"=FALSE, "Left Button 3"=FALSE} ("Left Buttons")) -> ()
                  n119 = local write "ATM Messages"("Your session has been terminated due to inactivity or menu selection. \n\nPlease take your card\n\nGoodbye!" ("ATM")) -> ()
                  n120 = property on="Right Menu" class="Clust (strict)"("DisabledEnum"=w392) -> ()  [unwired: 2 in, 2 out]
                  n121 = property on="Right Buttons" class="Clust (strict)"("DisabledEnum"=w392) -> ()  [unwired: 2 in, 2 out]
                  n122 = property on="Left Buttons" class="Clust (strict)"("DisabledEnum"=w392) -> ()  [unwired: 2 in, 2 out]
                  n123 = property on="Left Menu" class="Clust (strict)"("DisabledEnum"=w392) -> ()  [unwired: 2 in, 2 out]
                  n124 = call "ClientTCPIP.vi"("timeout \nms (60000)"=60000 ("timeout ms (60000)"), "port"=u16 1103 ("remote port or service name"), "Input String"="Halt?Halt" ("data in")) -> ("error out"=→"Exit Error":errorcluster)  [unwired: 7 in, 1 out]
                }
                event "Right Buttons.Right Button 1": Value Change {
                  w409 = T7."Enabled" ("Disabled")
                  # "Assigns the value 'Deposit' to the enumeration variable named 'Events', \nand proceeds upon pressing the enter button"
                  # "Component Properties"
                  # "Enable the deposit of a specified amount \nof cash into the user's account"
                  n125 = event-data() -> ()  [unwired: 1 in, 6 out]
                  n126 = property on="User Input" class="Str"("DisabledEnum"=w409, "Key Focus"=TRUE) -> ()  [unwired: 2 in, 2 out]
                  n127 = property on="Enter Button" class="Bool (strict)"("DisabledEnum"=w409) -> ()  [unwired: 2 in, 2 out]
                  n128 = local write "ATM Messages"("Please enter amount to deposit \nand press Enter (E) when done" ("ATM - Brank")) -> ()
                  n129 = local write "Right Buttons"(T1 {"Right Button 1"=FALSE, "Right Button 2"=FALSE, "Right Button 3"=FALSE} ("Right Buttons")) -> ()
                  n130 = local write "Events"(ControllerAccount."Deposit" ("Enter")) -> ()
                }
                event "Right Buttons.Right Button 2": Value Change {
                  w417 = T7."Enabled" ("Disabled")
                  # "Assigns the value 'Deposit' to the enumeration variable named 'Events', \nand proceeds upon pressing the enter button"
                  # "Enable the withdrawal of a specified amount \nof cash out of user's account"
                  # "Component Properties"
                  n131 = event-data() -> ()  [unwired: 1 in, 6 out]
                  n132 = local write "ATM Messages"("Please enter amount to withdraw \nand press Enter (E) when done" ("ATM - Brank")) -> ()
                  n133 = local write "Right Buttons"(T1 {"Right Button 1"=FALSE, "Right Button 2"=FALSE, "Right Button 3"=FALSE} ("Right Buttons")) -> ()
                  n134 = property on="User Input" class="Str"("DisabledEnum"=w417, "Key Focus"=TRUE) -> ()  [unwired: 2 in, 2 out]
                  n135 = property on="Enter Button" class="Bool (strict)"("DisabledEnum"=w417) -> ()  [unwired: 2 in, 2 out]
                  n136 = local write "Events"(ControllerAccount."Withdraw" ("Enter")) -> ()
                }
                event "Right Buttons.Right Button 3": Value Change {
                  w420 = T7."Disabled and Grayed Out" ("Disabled")
                  # "This button serves the purpose of facilitating the withdrawal \nof a predetermined amount of cash"
                  # "Process"
                  # "Component Properties"
                  n137 = event-data() -> ()  [unwired: 1 in, 6 out]
                  n138 = call "EventListener.vi"("Account No."=w419, "Cases"="User/FastCash") -> ()  [unwired: 10 in]
                  n139 = property on="Right Menu" class="Clust (strict)"("DisabledEnum"=w420) -> ()  [unwired: 2 in, 2 out]
                  n140 = property on="Right Buttons" class="Clust (strict)"("DisabledEnum"=w420) -> ()  [unwired: 2 in, 2 out]
                  n141 = property on="Left Buttons" class="Clust (strict)"("DisabledEnum"=w420) -> ()  [unwired: 2 in, 2 out]
                  n142 = property on="Left Menu" class="Clust (strict)"("DisabledEnum"=w420) -> ()  [unwired: 2 in, 2 out]
                  n143 = local write "ATM Messages"("Processing..." ("ATM Messages")) -> ()
                  n144 = local write "Right Buttons"(T1 {"Right Button 1"=FALSE, "Right Button 2"=FALSE, "Right Button 3"=FALSE} ("Right Buttons")) -> ()
                  n145 = local read "Account No."() -> (w434:string)
                  n146 = Concatenate Strings "Concatenate \nStrings"(w434, "?" ("string"), "Withdraw" ("string"), "?" ("string"), "50" ("string")) -> (w425:string)
                  n147 = call "ClientTCPIP.vi"("timeout \nms (60000)"=60000 ("timeout ms (60000)"), "port"=u16 1103 ("remote port or service name"), "Input String"=w425) -> ("error out"=→"Fast Cash \nWithdrawal Error":errorcluster, "Output Data"=w422:string)  [unwired: 7 in]
                  n148 = xnode "Match Regular Expression"("input string"=w422, "regular expression"="\\?") -> ("before match"=w426:string)  [unwired: 4 in, 4 out]
                  n149 = case shown="\"True\", Default" w426 {
                    frame "False" {
                      n150 = local write "ATM Messages"("There are insufficient funds in your account. \nWe kindly request you to verify your balance and attempt the transaction again." ("ATM - Brank")) -> ()
                    }
                    frame "True", Default {
                      n151 = flat-sequence {
                        frame #0 {
                          n152 = local write "ATM Messages"("The withdrawal of $50 has been completed successfully." ("ATM - Brank")) -> ()
                          n153 = Wait (ms)(milliseconds to wait=u32 1000) -> ()  [unwired: 1 out]
                        }
                        frame #1 {
                          n154 = local read "Account No."() -> (w441:string)
                          n155 = call "Receipt.vi"("Account Number"=w441, "Value"="50", "Operation"="Withdrawn") -> ("Output"=w440:string)  [unwired: 8 in]
                          n156 = local write "ATM Messages"(w440) -> ()
                        }
                      }
                    }
                  }
                }
                event "Enter Button": Value Change {
                  # "Three events: Deactivate, Deposit, Withdraw"
                  n157 = event-data() -> ()  [unwired: 1 in, 6 out]
                  n158 = local write "Enter Button"(FALSE ("Enter Button")) -> ()
                  n159 = local read "Events"() -> (w564:T5)
                  n160 = case shown="\"Withdraw\"" w564 {
                    tunnel: w561 -> [_ w566 w736]
                    frame "Deactivate", Default {
                      # "Initial State"
                    }
                    frame "Deposit" {
                      (unwired) 5 ("y")
                      # "Verify whether the user has entered any integer value by evaluating the length of the string"
                      n161 = local read "User Input"() -> (w577:string)
                      n162 = call <vilib>:"Trim Whitespace.vi"("string"=w577) -> ("trimmed string"=w568:string)  [unwired: 1 in]
                      n163 = Match Pattern "Match \nPattern"(string=w568, regular expression="[0-9]+") -> (before substring=w574:string, after substring=w573:string)  [unwired: 1 in, 2 out]
                      n164 = String Length(string=w568) -> (length=w578:i32)
                      n165 = String Length(string=w574) -> (length=w576:i32)
                      n166 = String Length(string=w573) -> (length=w575:i32)
                      n167 = Not Equal To 0?(x=w578) -> (x != 0?=w579:bool)
                      n168 = Equal To 0?(x=w576) -> (x = 0?=w572:bool)
                      n169 = Equal To 0?(x=w575) -> (x = 0?=w571:bool)
                      n170 = And(x=w572, y=w571) -> (x .and. y?=w570:bool)
                      n171 = And(x=w579, y=w570) -> (x .and. y?=w567:bool)
                      n172 = case shown="False" w567 {
                        tunnel: w568 -> [_ w594]
                        tunnel: w566 -> [w581 _]
                        frame False {
                          n173 = call "EventListener.vi"("Account No."=w581, "Cases"="User/Deposit/Invalid") -> ()  [unwired: 10 in]
                          n174 = local write "ATM Messages"("The input provided is invalid.\n \nWe kindly ask you to verify your balance and attempt the transaction again." ("ATM - Brank")) -> ()
                        }
                        frame True {
                          w584 = T7."Disabled and Grayed Out" ("Disabled")
                          # "This event represents the fundamental logic behind the deposit function"
                          # "Component Properties"
                          # "Process"
                          n175 = property on="Right Menu" class="Clust (strict)"("DisabledEnum"=w584) -> ()  [unwired: 2 in, 2 out]
                          n176 = property on="Right Buttons" class="Clust (strict)"("DisabledEnum"=w584) -> ()  [unwired: 2 in, 2 out]
                          n177 = property on="Left Buttons" class="Clust (strict)"("DisabledEnum"=w584) -> ()  [unwired: 2 in, 2 out]
                          n178 = property on="Left Menu" class="Clust (strict)"("DisabledEnum"=w584) -> ()  [unwired: 2 in, 2 out]
                          n179 = local write "ATM Messages"("Processing..." ("ATM Messages")) -> ()
                          n180 = local read "Account No."() -> (w583:string)
                          n181 = Concatenate Strings "Concatenate \nStrings"(w583, "?" ("string"), "Deposit" ("string"), "?" ("string"), w594) -> (w589:string)
                          n182 = call "ClientTCPIP.vi"("timeout \nms (60000)"=60000 ("timeout ms (60000)"), "port"=u16 1103 ("remote port or service name"), "Input String"=w589) -> ("error out"=→"Deposit Error":errorcluster, "Output Data"=w586:string)  [unwired: 7 in]
                          n183 = xnode "Match Regular \nExpression"("input string"=w586, "regular expression"="\\?") -> ("before match"=w593:string, "after match"=w592:string)  [unwired: 4 in, 3 out]
                          n184 = case shown="\"False\"" w593 {
                            tunnel: w592 -> [_ w721]
                            tunnel: w583 -> [w715 w719]
                            frame "False" {
                              n185 = call "EventListener.vi"("Account No."=w715, "Cases"="User/OutOfRange") -> ()  [unwired: 10 in]
                              n186 = local write "ATM Messages"("The validation did not pass due to either \ninsufficient account authorization or the deposit amount falling outside \nthe range of 20 to 2000" ("ATM Messages")) -> ()
                            }
                            frame "True", Default {
                              n187 = flat-sequence {
                                tunnel: w721 -> [w723]
                                tunnel: [w723] -> w720
                                tunnel: w719 -> [w722]
                                tunnel: [w722] -> w718
                                tunnel: w720 -> [w729]
                                tunnel: w718 -> [w728]
                                frame #0 {
                                n188 = Concatenate Strings("$ " ("string"), w723, "\nDeposited" ("string")) -> (w727:string)
                                n189 = local write "ATM Messages"(w727) -> ()
                                n190 = Wait (ms)(milliseconds to wait=u32 1000) -> ()  [unwired: 1 out]
                                }
                                frame #1 {
                                n191 = local read "User Input"() -> (w733:string)
                                n192 = local read "Account No."() -> (w732:string)
                                n193 = call "EventListener.vi"("Amount"=w729, "Account No."=w728, "Cases"="User/Deposit/True") -> ()  [unwired: 9 in]
                                n194 = call "Receipt.vi"("Account Number"=w732, "Value"=w733, "Operation"="Deposited") -> ("Output"=w734:string)  [unwired: 8 in]
                                n195 = local write "ATM Messages"(w734) -> ()
                                }
                              }
                            }
                          }
                        }
                      }
                    }
                    frame "Withdraw" {
                      (unwired) 5 ("y")
                      # "Verify whether the user has entered any integer value by evaluating the length of the string"
                      n196 = local read "User Input"() -> (w747:string)
                      n197 = call <vilib>:"Trim Whitespace.vi"("string"=w747) -> ("trimmed string"=w737:string)  [unwired: 1 in]
                      n198 = Match Pattern "Match \nPattern"(string=w737, regular expression="[0-9]+") -> (before substring=w744:string, after substring=w743:string)  [unwired: 1 in, 2 out]
                      n199 = String Length(string=w737) -> (length=w748:i32)
                      n200 = String Length(string=w744) -> (length=w746:i32)
                      n201 = String Length(string=w743) -> (length=w745:i32)
                      n202 = Not Equal To 0?(x=w748) -> (x != 0?=w749:bool)
                      n203 = Equal To 0?(x=w746) -> (x = 0?=w742:bool)
                      n204 = Equal To 0?(x=w745) -> (x = 0?=w741:bool)
                      n205 = call "EventListener.vi"("Account No."=w736, "Cases"="User/Invalid") -> ()  [unwired: 10 in]
                      n206 = And(x=w742, y=w741) -> (x .and. y?=w740:bool)
                      n207 = And(x=w749, y=w740) -> (x .and. y?=w738:bool)
                      n208 = case shown="False" w738 {
                        tunnel: w737 -> [_ w762]
                        frame False {
                          n209 = local write "ATM Messages"("The input provided is invalid. \n\nWe kindly ask you to verify your balance and attempt the transaction again." ("ATM - Brank")) -> ()
                        }
                        frame True {
                          w752 = T7."Disabled and Grayed Out" ("Disabled")
                          # "This event represents the fundamental logic behind the withdraw function"
                          # "Component Properties"
                          # "Process"
                          n210 = property on="Right Menu" class="Clust (strict)"("DisabledEnum"=w752) -> ()  [unwired: 2 in, 2 out]
                          n211 = property on="Right Buttons" class="Clust (strict)"("DisabledEnum"=w752) -> ()  [unwired: 2 in, 2 out]
                          n212 = property on="Left Buttons" class="Clust (strict)"("DisabledEnum"=w752) -> ()  [unwired: 2 in, 2 out]
                          n213 = property on="Left Menu" class="Clust (strict)"("DisabledEnum"=w752) -> ()  [unwired: 2 in, 2 out]
                          n214 = local write "ATM Messages"("Processing..." ("ATM Messages")) -> ()
                          n215 = local read "Account No."() -> (w751:string)
                          n216 = Concatenate Strings "Concatenate\nStrings"(w751, "?" ("string"), "Withdraw" ("string"), "?" ("string"), w762) -> (w757:string)
                          n217 = call "ClientTCPIP.vi"("timeout \nms (60000)"=60000 ("timeout ms (60000)"), "port"=u16 1103 ("remote port or service name"), "Input String"=w757) -> ("error out"=→"Withdrawal Error":errorcluster, "Output Data"=w754:string)  [unwired: 7 in]
                          n218 = xnode "Match Regular \nExpression"("input string"=w754, "regular expression"="\\?") -> ("before match"=w760:string, "after match"=w759:string)  [unwired: 4 in, 3 out]
                          n219 = case shown="\"False\"" w760 {
                            tunnel: w759 -> [_ w889]
                            tunnel: w751 -> [w884 w886]
                            frame "False" {
                              n220 = call "EventListener.vi"("Account No."=w884, "Cases"="User/OutOfRange") -> ()  [unwired: 10 in]
                              n221 = local write "ATM Messages"("To ensure compliance, the minimum required account balance is 20, and the maximum allowable withdrawal amount is 2000." ("ATM - Brank")) -> ()
                            }
                            frame "True", Default {
                              n222 = flat-sequence {
                                tunnel: w889 -> [w891]
                                tunnel: [w891] -> w888
                                tunnel: [w890] -> w887
                                tunnel: w886 -> [w890]
                                tunnel: w888 -> [w897]
                                tunnel: w887 -> [w896]
                                frame #0 {
                                n223 = Concatenate Strings "Concatenate\nStrings"("$ " ("string"), w891, "\nWithdrawn" ("string")) -> (w895:string)
                                n224 = local write "ATM Messages"(w895) -> ()
                                n225 = Wait (ms)(milliseconds to wait=u32 1000) -> ()  [unwired: 1 out]
                                }
                                frame #1 {
                                n226 = local read "User Input"() -> (w900:string)
                                n227 = local read "Account No."() -> (w899:string)
                                n228 = call "Receipt.vi"("Account Number"=w899, "Value"=w900, "Operation"="Withdrawn") -> ("Output"=w902:string)  [unwired: 8 in]
                                n229 = call "EventListener.vi"("Amount"=w897, "Account No."=w896, "Cases"="User/Withdraw/True") -> ()  [unwired: 9 in]
                                n230 = local write "ATM Messages"(w902) -> ()
                                }
                              }
                            }
                          }
                        }
                      }
                    }
                  }
                }
              }
            }
          }
          n231 = Or(x=w342, y=FALSE) -> (x .or. y?=w340:bool)
        }
      }
    }
  }
